vi "2010_FireEveryLastFridayOfMonth.vi"(8 "error in (no error)":errorcluster) -> (0 "error out":errorcluster)   [LabVIEW 2013]
uses:
  source/Cron.Jenkins/Cron.Jenkins.lvclass/Cron.Jenkins.ctl
  source/Cron.Jenkins/Write Job Name.vi
  <vilib>/addons/_JKI Toolkits/Caraya/classes/Assert/Assert True.vi
  source/Cron/Create Cron Job.vi
  source/Cron/Compute Next Cron.vi
  source/Cron.Jenkins/Cron.Jenkins.lvclass
  <vilib>/addons/_JKI Toolkits/Caraya/classes/Test/Test.lvclass
  <vilib>/addons/_JKI Toolkits/Caraya/classes/Assert/Assert.lvclass
  source/openCron.lvlib
panel:
  out "Occurences":timestamp[](array[timestamp])
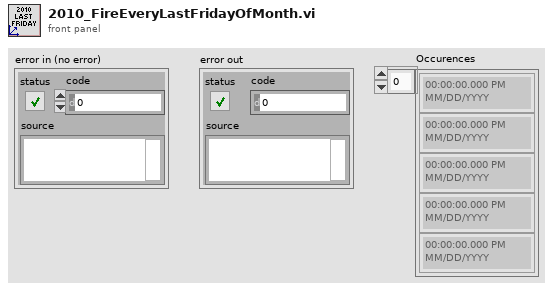
[diagram p1: front panel]
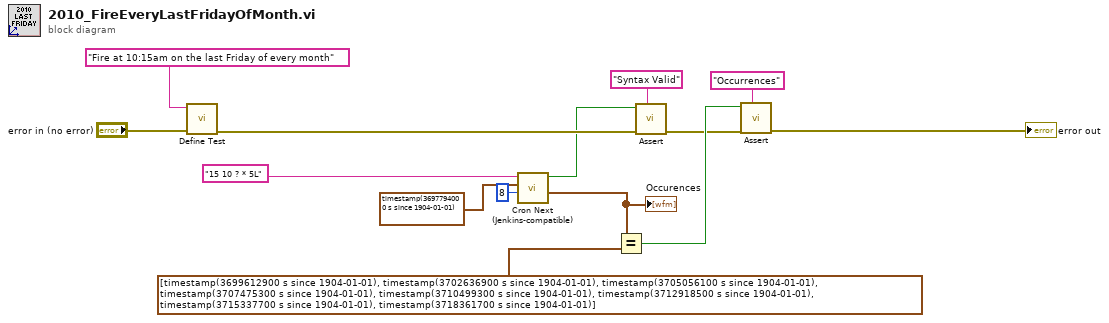
[diagram p0: block diagram]
diagram:
  n1 = call <vilib>:"Define Test.vi"("error in (no error)"="error in (no error)", "Label (VI Title)"="Fire at 10:15am on the last Friday of every month") -> ("error out"=w11:errorcluster)  [unwired: 9 in]
  n2 = call "Cron Next (Jenkins-compatible).vi"("Nb Occurences (min: 1)"=u16 8, "Reference timestamp (Now)"=timestamp(3697794000 s since 1904-01-01) ("y"), "Cron Expression"="15 10 ? * 5L" ("Expression")) -> ("Occurences"=w7:timestamp[], "syntax valid?"=w8:bool)  [unwired: 6 in, 1 out]
  "Occurences" <- w7
  n3 = Equal?(x=w7, y=timestamp[] [timestamp(3699612900 s since 1904-01-01), timestamp(3702636900 s since 1904-01-01), timestamp(3705056100 s since 1904-01-01), timestamp(3707475300 s since 1904-01-01), timestamp(3710499300 s since 1904-01-01), timestamp(3712918500 s since 1904-01-01), timestamp(3715337700 s since 1904-01-01), timestamp(3718361700 s since 1904-01-01)]) -> (x = y?=w10:bool)
  n4 = call-poly <vilib>:"Assert.vi"("Label"="Syntax Valid" ("Label (VI Title)"), "error in (no error)"=w11, "True?"=w8) -> ("error out"=w9:errorcluster)  [unwired: 8 in]
  n5 = call-poly <vilib>:"Assert.vi"("Label"="Occurrences" ("Label (VI Title)"), "error in (no error)"=w9, "True?"=w10) -> ("error out"=→"error out":errorcluster)  [unwired: 8 in]
